vi "Close.vi"(8 "error in (no error)":errorcluster, 10 "Exit Code (0)":i32, 11 "CLI in":refnum<class "CLI.lvclass">) -> ()   [LabVIEW 2016, in "Script.lvlib"]
uses:
  Script.lvlib
  <vilib>/Wiresmith Technology/G CLI/CLI Class/CLI.lvclass
  <vilib>/Utility/error.llb/DialogType.ctl
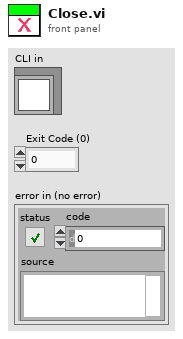
[diagram p1: front panel]
types:
  T1 = typedef "DialogType.ctl" = u16
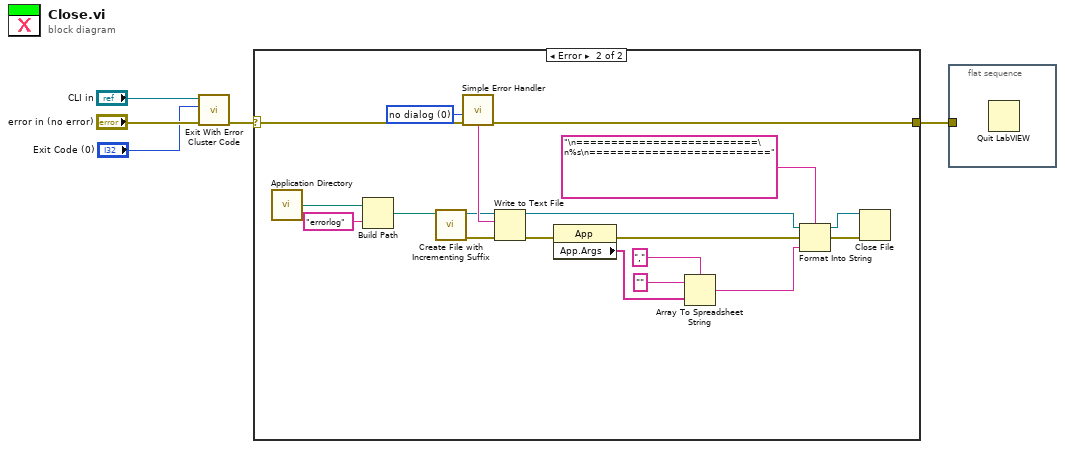
[diagram p0: block diagram]
diagram:
  n1 = call <vilib>:"Exit With Error Cluster Code.vi"("error in (no error)"="error in (no error)", "No Error Code (0)"="Exit Code (0)", "CLI in"="CLI in") -> ("error out"=w2:errorcluster)  [unwired: 8 in]
  n2 = case shown="Error" w2 {
    selector: w2 -> [w6 w25]
    tunnel: [w6 w24] -> w1
    frame No Error {
    }
    frame Error {
      w22 = T1 0 items=["no dialog", "OK message", "continue or stop message", "OK message + warnings", "continue/stop + warnings"] ("type of dialog (OK msg:1)")
      n3 = call <vilib>:"Application Directory.vi"() -> ("Application Directory"=w19:path)
      n4 = Build Path(base path=w19, name or relative path="errorlog") -> (appended path=w18:path)
      n5 = call <vilib>:"Create File with Incrementing Suffix.vi"("file path"=w18) -> ("error out"=w21:errorcluster, "refnum out"=w20:refnum<file>)  [unwired: 8 in, 1 out]
      n6 = call <vilib>:"Simple Error Handler.vi"("type of dialog (OK msg:1)"=w22, "error in (no error)"=w25) -> ("error out"=w24:errorcluster, "message"=w23:string)  [unwired: 3 in, 3 out]
      n7 = Write to Text File(file (use dialog)=w20, text=w23, error in=w21) -> (refnum out=w10:refnum<file>, error out=w16:errorcluster)  [unwired: 1 in, 1 out]
      n8 = property class="App"(error in=w16) -> (error out=w13:errorcluster, "App.Args"=w15:string[])  [unwired: 1 in, 1 out]
      n9 = Array To Spreadsheet String(delimiter (Tab)=",", array=w15, 3:"" ("format string")) -> (spreadsheet string=w8:string)
      n10 = Format Into String(format string="\n==========================\n%s\n==========================", initial string=w10, error in=w13, w8) -> (resulting string=w11:refnum<file>, error out=w12:errorcluster)
      n11 = Close File(refnum=w11, error in=w12) -> ()  [unwired: 2 out]
    }
  }
  n12 = flat-sequence {
    tunnel: w1 -> [_]
    frame #0 {
      n13 = Quit LabVIEW() -> ()  [unwired: 1 in]
    }
  }
